vi "Raise Error for Failed VI Updates.vi"(8 "error in":errorcluster, 11 "Failed VIs":string[](array[string])) -> (0 "error out":errorcluster)   [LabVIEW 2019, in "Engine.lvclass"]
uses:
  Engine.lvclass
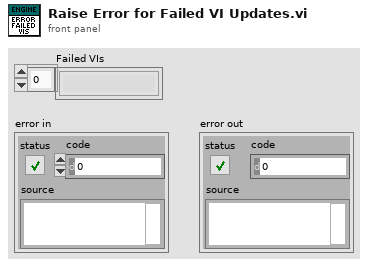
[diagram p1: front panel]
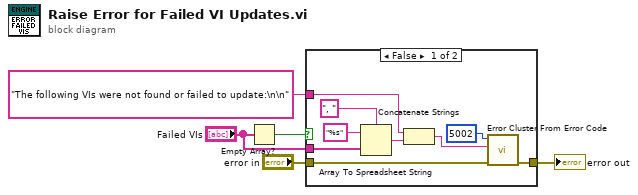
[diagram p0: block diagram]
diagram:
  n1 = Empty Array?(array="Failed VIs") -> (empty?=w1:bool)
  n2 = case shown="False" w1 {
    tunnel: "Failed VIs" -> [w13 _]
    tunnel: [w11 w15] -> w5
    tunnel: "error in" -> [w10 w15]
    tunnel: "The following VIs were not found or failed to update:\n\n" ("string") -> [w6 _]
    frame False {
      n3 = Array To Spreadsheet String(delimiter (Tab)=", ", array=w13, 3:"%s" ("format string")) -> (spreadsheet string=w12:string)
      n4 = Concatenate Strings(w6, w12) -> (w7:string)
      n5 = call <vilib>:"Error Cluster From Error Code.vi"("error in (no error)"=w10, "error message (\"\")"=w7, "error code (0)"=5002) -> ("error out"=w11:errorcluster)  [unwired: 6 in]
    }
    frame True {
    }
  }
  "error out" <- w5
